vi "Test Server-Client SSL.vi"() -> ()   [LabVIEW 2020]
uses:
  <vilib>/LabVIEW Open Source Project/MQTT Client/Client class/Client.lvclass/Client.ctl
  <vilib>/LabVIEW Open Source Project/MQTT Connection/MQTT_Base/Base Class/MQTT_Base.lvclass/MQTT_Base.ctl
  <vilib>/LabVIEW Open Source Project/MQTT Broker/Server class/Server.lvclass/Server.ctl
  source/Connection.SecuredTCP/Connection.TCP-TLS.lvclass
  C:/Program Files (x86)/National Instruments/LabVIEW 2020/vi.lib/LabVIEW Open Source Project/MQTT Connection/MQTT_Connection/Connection/Connection.lvclass
  <vilib>/LabVIEW Open Source Project/MQTT Broker/Server class/Server.lvclass
  C:/Program Files (x86)/National Instruments/LabVIEW 2020/vi.lib/LabVIEW Open Source Project/MQTT Connection/MQTT_Base/Base Class/MQTT_Base.lvclass
  <vilib>/LabVIEW Open Source Project/MQTT Client/Client class/Client.lvclass
  <vilib>/LabVIEW Open Source Project/MQTT Control Packets/Control Packets/PUBLISH/PUBLISH.lvclass
  <vilib>/LabVIEW Open Source Project/MQTT Connection/MQTT_Base/Base Class/MQTT_Base.lvclass
  <vilib>/LabVIEW Open Source Project/MQTT Control Packets/Control Packets/ControlPacket/ControlPacket.lvclass
  C:/Program Files (x86)/National Instruments/LabVIEW 2020/vi.lib/LabVIEW Open Source Project/MQTT Control Packets/Control Packets/ControlPacket/ControlPacket.lvclass
panel:
  out "error client 2":errorcluster
  out "error client 1":errorcluster
  in  "publish period (ms)":i32=100 min=1 max=5000
  in  "Unsubscribe":bool
  out "Unsuback":bool
  out "Waveform Chart":dbl(graph)
  in  "Subscribe":bool
  out "Suback":bool
  out "NbConnections":u32
  out "error server":errorcluster
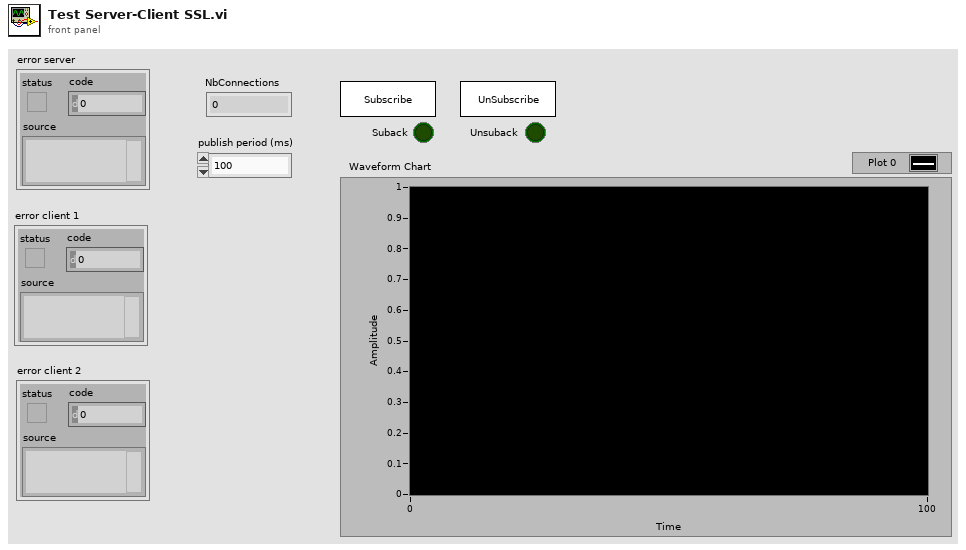
[diagram p1: front panel]
types:
  T1 = typedef "MQTT Client.lvlib/Client.lvclass/Public Events -- cluster.ctl" = cluster{"Connection Status":refnum<user-event>, "Connected":refnum<user-event>, "Application Message":refnum<user-event>}
  T2 = typedef "MQTT Base.lvlib/MQTT_Base.lvclass/Public Events -- cluster.ctl" = cluster{"Stop Event":refnum<user-event>, "Error Event":refnum<user-event>, "Inbound Message":refnum<user-event>}
  T3 = typedef "MQTT Server.lvlib/Server.lvclass/Public Events -- cluster.ctl" = cluster{"NbConnections":refnum<user-event>}
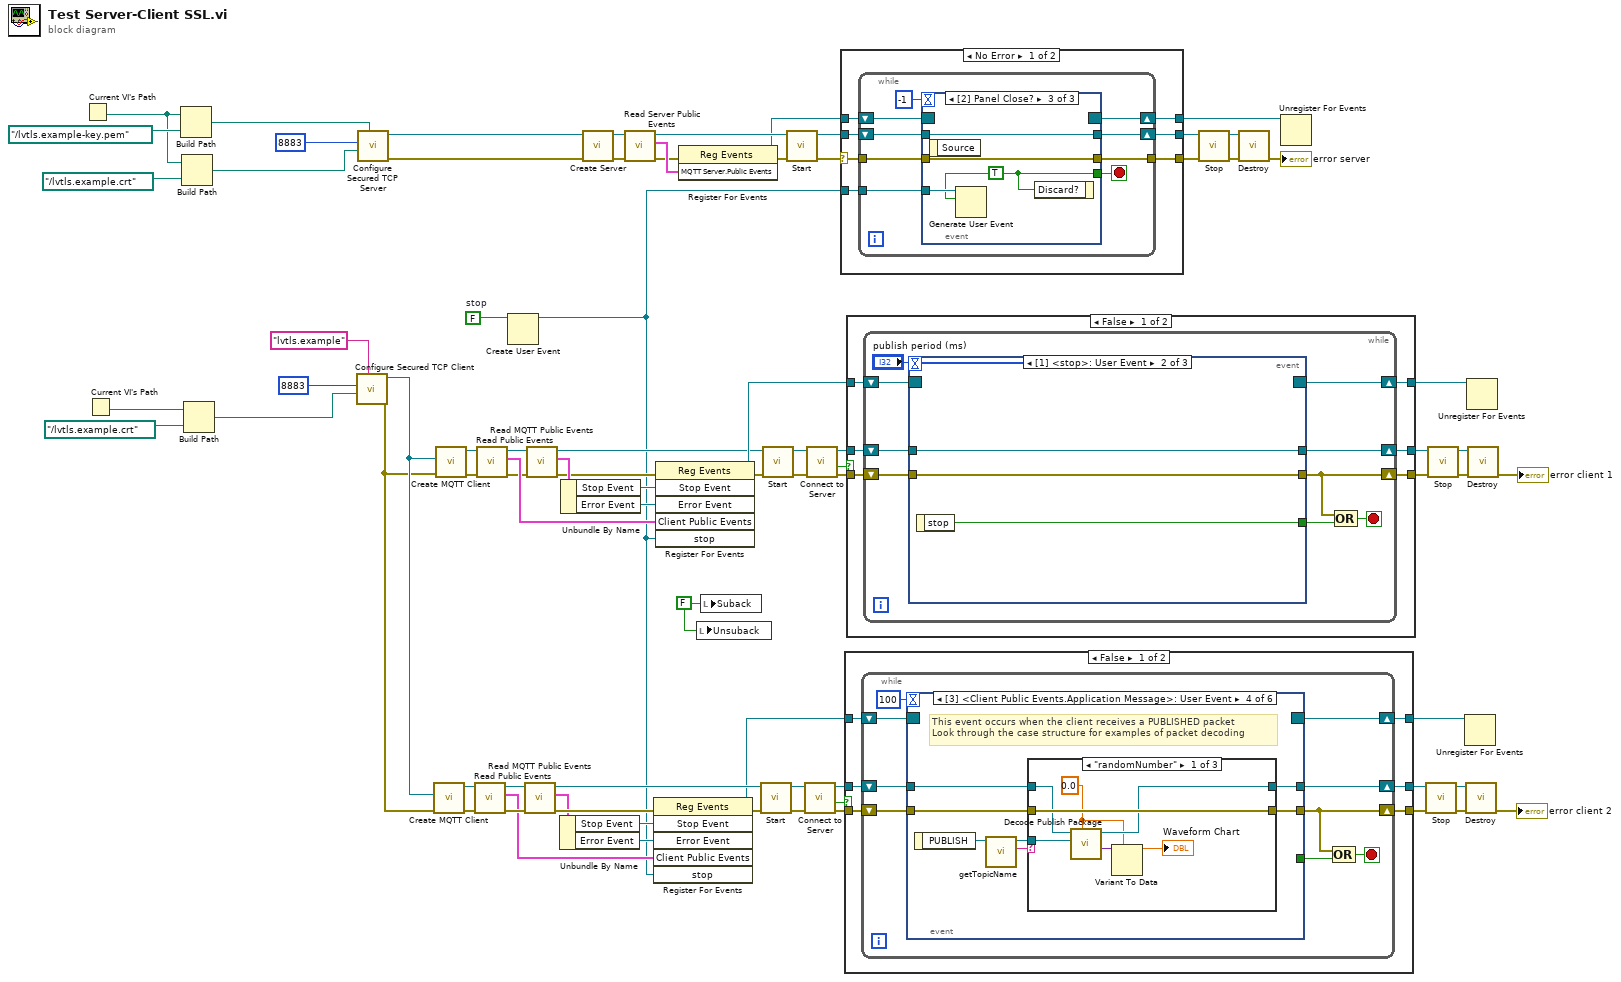
[diagram p0: block diagram]
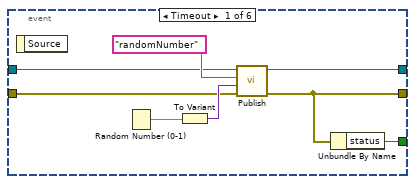
[diagram p2: hidden frame]
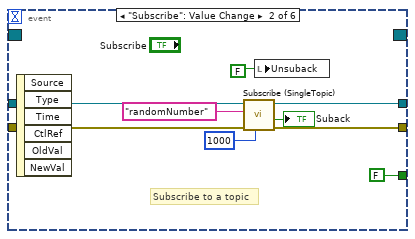
[diagram p3: hidden frame]
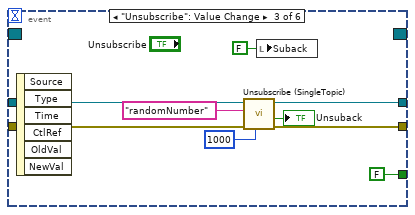
[diagram p4: hidden frame]
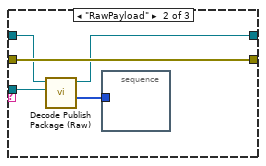
[diagram p5: hidden frame]
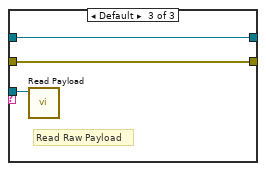
[diagram p6: hidden frame]
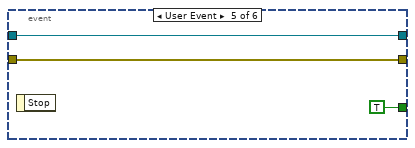
[diagram p7: hidden frame]
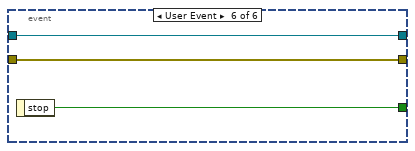
[diagram p8: hidden frame]
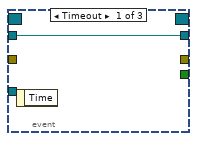
[diagram p10: hidden frame]
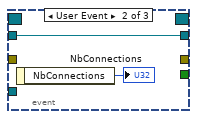
[diagram p11: hidden frame]
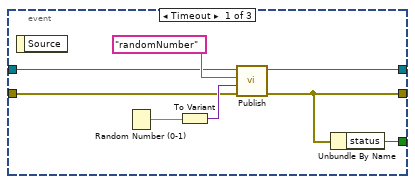
[diagram p13: hidden frame]
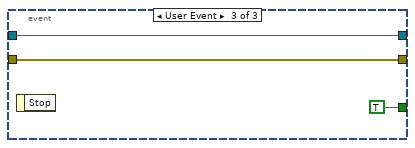
[diagram p14: hidden frame]
diagram:
  w19 = FALSE  # stop
  w20 = FALSE ("Suback")
  n1 = Current VI's Path() -> (path=w8:path)
  n2 = Current VI's Path() -> (path=w5:path)
  n3 = Build Path(base path=w8, name or relative path=path "../lvtls.example-key.pem" ("Server private key")) -> (appended path=w7:path)
  n4 = Build Path(base path=w8, name or relative path=path "../lvtls.example.crt" ("X.509 Certificate")) -> (appended path=w6:path)
  n5 = Build Path(base path=w5, name or relative path=path "../lvtls.example.crt" ("Server private key")) -> (appended path=w3:path)
  n6 = call "Configure Secured TCP Client.vi"("Hostname"="lvtls.example", "X.509 Certificate"=w3, "remote port (443)"=u16 8883 ("remote port (80)")) -> ("error out"=w11:errorcluster, "Secured TCP Connection"=w15:refnum<class "Connection.TCP-TLS.lvclass">)  [unwired: 6 in, 1 out]
  n7 = call "Configure Secured TCP Server.vi"("Server private key"=w7, "X.509 Certificate"=w6, "remote port (443)"=u16 8883 ("remote port (80)")) -> ("error out"=w12:errorcluster, "Secured TCP Connection"=w14:refnum<class "Connection.TCP-TLS.lvclass">)  [unwired: 6 in, 1 out]
  n8 = call <vilib>:"Create MQTT Client.vi"("error in (no error)"=w11, "Connection Configuration"=w15) -> ("error out"=w40:errorcluster, "Client out"=w42:refnum<class "Client.lvclass">)  [unwired: 8 in]
  n9 = call <vilib>:"Create MQTT Client.vi"("error in (no error)"=w11, "Connection Configuration"=w15) -> ("error out"=w60:errorcluster, "Client out"=w58:refnum<class "Client.lvclass">)  [unwired: 8 in]
  n10 = call <vilib>:"Read Public Events.vi"("error in (no error)"=w40, "Client in"=w42) -> ("error out"=w39:errorcluster, "Client Public Events"=w37:T1, "Client out"=w41:refnum<class "Client.lvclass">)  [unwired: 7 in]
  n11 = call <vilib>:"Read Public Events.vi"("error in (no error)"=w60, "Client in"=w58) -> ("error out"=w61:errorcluster, "Client Public Events"=w63:T1, "Client out"=w59:refnum<class "Client.lvclass">)  [unwired: 7 in]
  n12 = Create User Event(user event datatype=w19) -> (user event=w18:refnum<user-event>)  [unwired: 1 in, 1 out]
  n13 = call <vilib>:"Read MQTT Public Events.vi"("error in (no error)"=w39, "MQTT_Base in"=w41) -> ("error out"=w38:errorcluster, "MQTT Public Events"=w25:T2, "MQTT_Base out"=w35:refnum<class "Client.lvclass">)  [unwired: 7 in]
  n14 = call <vilib>:"Read MQTT Public Events.vi"("error in (no error)"=w61, "MQTT_Base in"=w59) -> ("error out"=w62:errorcluster, "MQTT Public Events"=w75:T2, "MQTT_Base out"=w65:refnum<class "Client.lvclass">)  [unwired: 7 in]
  n15 = Unbundle By Name(w25) -> ("Stop Event"=w27:refnum<user-event>, "Error Event"=w26:refnum<user-event>)
  n16 = Unbundle By Name(w75) -> ("Stop Event"=w73:refnum<user-event>, "Error Event"=w74:refnum<user-event>)
  n17 = call <vilib>:"Create Server.vi"("error in (no error)"=w12, "Connection Configuration"=w14) -> ("error out"=w44:errorcluster, "Server"=w43:refnum<class "Server.lvclass">)  [unwired: 8 in]
  n18 = call <vilib>:"Read Server Public Events.vi"("error in (no error)"=w44, "Server in"=w43) -> ("error out"=w45:errorcluster, "MQTT Server.Public Events"=w46:T3, "Server out"=w49:refnum<class "Server.lvclass">)  [unwired: 7 in]
  n19 = register-events(error in=w38, w27, w26, w37, w18) -> (reference out=w32:refnum<event-registration>, error out=w36:errorcluster)  [unwired: 1 in]
  n20 = register-events(error in=w62, w73, w74, w63, w18) -> (reference out=w68:refnum<event-registration>, error out=w64:errorcluster)  [unwired: 1 in]
  n21 = register-events(error in=w45, w46) -> (reference out=w47:refnum<event-registration>, error out=w51:errorcluster)  [unwired: 1 in]
  n22 = local write "Unsuback"(w20) -> ()
  n23 = local write "Suback"(w20) -> ()
  n24 = call <vilib>:"Start.vi"("error in (no error)"=w36, "MQTT_Base in"=w35) -> ("error out"=w33:errorcluster, "MQTT_Base out"=w34:refnum<class "Client.lvclass">)  [unwired: 7 in, 1 out]
  n25 = call <vilib>:"Start.vi"("error in (no error)"=w64, "MQTT_Base in"=w65) -> ("error out"=w67:errorcluster, "MQTT_Base out"=w66:refnum<class "Client.lvclass">)  [unwired: 7 in, 1 out]
  n26 = call <vilib>:"Start.vi"("error in (no error)"=w51, "MQTT_Base in"=w49) -> ("error out"=w52:errorcluster, "MQTT_Base out"=w50:refnum<class "Server.lvclass">)  [unwired: 7 in, 1 out]
  n27 = call <vilib>:"Connect to Server.vi"("error in (no error)"=w33, "Client in"=w34) -> ("error out"=w29:errorcluster, "timed out"=w30:bool, "Client out"=w28:refnum<class "Client.lvclass">)  [unwired: 6 in, 1 out]
  n28 = call <vilib>:"Connect to Server.vi"("error in (no error)"=w67, "Client in"=w66) -> ("error out"=w71:errorcluster, "timed out"=w70:bool, "Client out"=w72:refnum<class "Client.lvclass">)  [unwired: 6 in, 1 out]
  n29 = case shown="No Error" w52 {
    selector: w52 -> [w81 w103]
    tunnel: w50 -> [w86 w105]
    tunnel: [w85 w105] -> w55
    tunnel: w47 -> [w84 w104]
    tunnel: [w83 w104] -> w48
    tunnel: [w82 w103] -> w57
    tunnel: w18 -> [w80 _]
    frame No Error {
      n30 = while {
        shift-right: [w92] -> w85
        shift-left: w86 -> [w94]
        tunnel: [w89] -> w82
        tunnel: w81 -> [w88]
        shift-right: [w90] -> w83
        shift-left: w84 -> [w91]
        tunnel: w80 -> [w87]
        stop <- w93 stop-if-true
        n31 = event shown="[2] Panel Close?" {
          selector: w91 -> [_ _ _]
          dyn-events: [_ _ _] -> w90
          timeout: -1 -> [_ _ _]
          tunnel: w94 -> [w96 w98 w102]
          tunnel: [_ _ w99] -> w93
          tunnel: [w96 w98 w102] -> w92
          tunnel: [_ _ w101] -> w89
          tunnel: w88 -> [_ _ w101]
          tunnel: w87 -> [_ _ w100]
          event Timeout {
            n32 = event-data() -> ()  [unwired: 1 in, 1 out]
          }
          event User Event {
            n33 = event-data() -> ("NbConnections"=→"NbConnections":u32)  [unwired: 1 in]
          }
          event Panel Close? {
            w99 = TRUE ("Discard?")
            n34 = event-data() -> ()  [unwired: 1 in, 1 out]
            n35 = Generate User Event(user event=w100, event data cluster=w99) -> ()  [unwired: 2 in, 2 out]
            n36 = event-data("Discard?"=w99) -> ()  [unwired: 1 in, 1 out]
          }
        }
      }
    }
    frame Error {
    }
  }
  n37 = case shown="False" w30 {
    tunnel: w32 -> [w111 w177]
    tunnel: [w110 w177] -> w31
    tunnel: w29 -> [w107 w175]
    tunnel: w28 -> [w109 w176]
    tunnel: [w108 w176] -> w23
    tunnel: [w106 w175] -> w21
    frame False {
      n38 = while {
        shift-right: [w119] -> w110
        shift-left: w111 -> [w120]
        shift-right: [w112] -> w108
        shift-left: w109 -> [w113]
        shift-right: [w117] -> w106
        shift-left: w107 -> [w118]
        stop <- w116 stop-if-true
        n39 = event shown="[3] <Client Public Events.Application Message>: User Event" {
          selector: w120 -> [_ _ _ _ _ _]
          dyn-events: [_ _ _ _ _ _] -> w119
          timeout: 100 -> [_ _ _ _ _ _]
          tunnel: w118 -> [w124 w135 w143 w148 w171 w174]
          tunnel: [w122 w134 w141 w149 w171 w174] -> w117
          tunnel: [w121 FALSE FALSE _ TRUE w172] -> w115
          tunnel: w113 -> [w125 w136 w145 w151 w169 w173]
          tunnel: [w123 w133 w144 w150 w169 w173] -> w112
          event Timeout {
            n40 = event-data() -> ()  [unwired: 1 in, 1 out]
            n41 = Random Number (0-1)() -> (number: 0 to 1=w127:dbl)
            n42 = To Variant(anything=w127) -> (Variant=w126:variant)
            n43 = call <vilib>:"Publish.vi"("error in (no error)"=w124, "Payload"=w126, "Topic Name (empty: Payload name)"="randomNumber", "Client in"=w125) -> ("error out"=w122:errorcluster, "Client out"=w123:refnum<class "Client.lvclass">)  [unwired: 5 in, 1 out]
            n44 = Unbundle By Name(w122) -> ("status"=w121:bool)
          }
          event "Subscribe": Value Change {
            # "Subscribe to a topic"
            n45 = event-data() -> ()  [unwired: 1 in, 6 out]
            n46 = call <vilib>:"Subscribe (SingleTopic).vi"("timeout (100ms)"=1000, "error in (no error)"=w135, "Topic Filter"="randomNumber" ("Topic Name (empty: Payload name)"), "MQTT_Base in"=w136) -> ("error out"=w134:errorcluster, "Ack"=→"Suback":bool, "MQTT_Base out"=w133:refnum<class "Client.lvclass">)  [unwired: 5 in]
            n47 = local write "Unsuback"(FALSE ("Suback")) -> ()
          }
          event "Unsubscribe": Value Change {
            n48 = event-data() -> ()  [unwired: 1 in, 6 out]
            n49 = call <vilib>:"Unsubscribe (SingleTopic).vi"("timeout (100ms)"=1000, "error in (no error)"=w143, "Topic Filter"="randomNumber" ("Topic Name (empty: Payload name)"), "MQTT_Base in"=w145) -> ("error out"=w141:errorcluster, "Ack"=→"Unsuback":bool, "MQTT_Base out"=w144:refnum<class "Client.lvclass">)  [unwired: 5 in]
            n50 = local write "Suback"(FALSE ("Suback")) -> ()
          }
          event User Event {
            # "This event occurs when the client receives a PUBLISHED packet\nLook through the case structure for examples of packet decoding"
            n51 = event-data() -> ("PUBLISH"=w153:refnum<class "PUBLISH.lvclass">)  [unwired: 1 in]
            n52 = call <vilib>:"getTopicName.vi"("PUBLISH in"=w153) -> ("Topic"=w152:string, "PUBLISH out"=w147:refnum<class "PUBLISH.lvclass">)  [unwired: 8 in, 1 out]
            n53 = case shown="\"randomNumber\"" w152 {
              tunnel: w151 -> [w158 w164 w168]
              tunnel: [w157 w162 w168] -> w150
              tunnel: [w160 w165 w167] -> w149
              tunnel: w148 -> [w160 w165 w167]
              tunnel: w147 -> [w159 w163 w166]
              frame "randomNumber" {
                w155 = 0.0 ("number (0 to 1)")
                n54 = call <vilib>:"Decode Publish Package.vi"("Type"=w155, "PUBLISH in"=w159, "MQTT_Base in"=w158) -> ("Payload"=w156:variant, "MQTT_Base out"=w157:refnum<class "Client.lvclass">)  [unwired: 5 in, 2 out]
                n55 = Variant To Data(type=w155, Variant=w156) -> (data=→"Waveform Chart":dbl)  [unwired: 1 in, 1 out]
              }
              frame "RawPayload" {
                n56 = call <vilib>:"Decode Publish Package (Raw).vi"("PUBLISH in"=w163, "MQTT_Base in"=w164) -> ("Payload"=w161:u8[], "MQTT_Base out"=w162:refnum<class "Client.lvclass">)  [unwired: 6 in, 2 out]
                n57 = stacked-sequence {
                  tunnel: w161 -> [_]
                  frame #0 {
                  }
                }
              }
              frame Default {
                # "Read Raw Payload"
                n58 = call <vilib>:"Read Payload.vi"("ControlPacket in"=w166) -> ()  [unwired: 9 in, 2 out]
              }
            }
          }
          event User Event {
            n59 = event-data() -> ()  [unwired: 1 in, 1 out]
          }
          event User Event {
            n60 = event-data() -> ("stop"=w172:bool)  [unwired: 1 in]
          }
        }
        n61 = Compound Arithmetic op=OR(w117, w115) -> (w116:bool)
      }
    }
    frame True {
    }
  }
  n62 = case shown="False" w70 {
    tunnel: w68 -> [w183 w209]
    tunnel: [w182 w209] -> w69
    tunnel: w71 -> [w179 w207]
    tunnel: w72 -> [w181 w208]
    tunnel: [w180 w208] -> w77
    tunnel: [w178 w207] -> w79
    frame False {
      n63 = while {
        shift-right: [w191] -> w182
        shift-left: w183 -> [w192]
        shift-right: [w184] -> w180
        shift-left: w181 -> [w185]
        shift-right: [w189] -> w178
        shift-left: w179 -> [w190]
        stop <- w188 stop-if-true
        n64 = event shown="[1] <stop>: User Event" {
          selector: w192 -> [_ _ _]
          dyn-events: [_ _ _] -> w191
          timeout: "publish period (ms)" -> [_ _ _]
          tunnel: w190 -> [w196 w202 w206]
          tunnel: [w194 w202 w206] -> w189
          tunnel: [w193 w201 TRUE] -> w187
          tunnel: w185 -> [w197 w203 w204]
          tunnel: [w195 w203 w204] -> w184
          event Timeout {
            n65 = event-data() -> ()  [unwired: 1 in, 1 out]
            n66 = Random Number (0-1)() -> (number: 0 to 1=w199:dbl)
            n67 = To Variant(anything=w199) -> (Variant=w198:variant)
            n68 = call <vilib>:"Publish.vi"("error in (no error)"=w196, "Payload"=w198, "Topic Name (empty: Payload name)"="randomNumber", "Client in"=w197) -> ("error out"=w194:errorcluster, "Client out"=w195:refnum<class "Client.lvclass">)  [unwired: 5 in, 1 out]
            n69 = Unbundle By Name(w194) -> ("status"=w193:bool)
          }
          event User Event {
            n70 = event-data() -> ("stop"=w201:bool)  [unwired: 1 in]
          }
          event User Event {
            n71 = event-data() -> ()  [unwired: 1 in, 1 out]
          }
        }
        n72 = Compound Arithmetic op=OR(w189, w187) -> (w188:bool)
      }
    }
    frame True {
    }
  }
  n73 = call <vilib>:"Stop.vi"("error in (no error)"=w57, "MQTT_Base in"=w55) -> ("error out"=w56:errorcluster, "MQTT_Base out"=w54:refnum<class "Server.lvclass">)  [unwired: 7 in, 1 out]
  n74 = call <vilib>:"Destroy.vi"("error in (no error)"=w56, "MQTT_Base in"=w54) -> ("error out"=→"error server":errorcluster)  [unwired: 8 in, 1 out]
  n75 = Unregister For Events(event registration refnum=w48) -> ()  [unwired: 1 in, 1 out]
  n76 = call <vilib>:"Stop.vi"("error in (no error)"=w21, "MQTT_Base in"=w23) -> ("error out"=w22:errorcluster, "MQTT_Base out"=w24:refnum<class "Client.lvclass">)  [unwired: 7 in, 1 out]
  n77 = call <vilib>:"Stop.vi"("error in (no error)"=w79, "MQTT_Base in"=w77) -> ("error out"=w78:errorcluster, "MQTT_Base out"=w76:refnum<class "Client.lvclass">)  [unwired: 7 in, 1 out]
  n78 = Unregister For Events(event registration refnum=w31) -> ()  [unwired: 1 in, 1 out]
  n79 = call <vilib>:"Destroy.vi"("error in (no error)"=w22, "MQTT_Base in"=w24) -> ("error out"=→"error client 2":errorcluster)  [unwired: 8 in, 1 out]
  n80 = Unregister For Events(event registration refnum=w69) -> ()  [unwired: 1 in, 1 out]
  n81 = call <vilib>:"Destroy.vi"("error in (no error)"=w78, "MQTT_Base in"=w76) -> ("error out"=→"error client 1":errorcluster)  [unwired: 8 in, 1 out]
